vi "Measure Current.vi"(8 "error in":errorcluster, 11 "4124 in":refnum<class "4124.lvclass">) -> (0 "error out":errorcluster, 2 "Current":dbl, 3 "4124 out":refnum<class "4124.lvclass">)   [LabVIEW 2018, in "4124.lvlib" / "4124.lvclass"]
uses:
  4124.lvclass
  <instrlib>/NI RMX-412x Power Supplies/NI RMX-412x Power Supplies.lvlib
  builds/Power_Supply.lvlibp/Power Supply.lvclass
  C:/Users/Ron.Dexter.LUMINARTECH/Desktop/builds/Power_Supply.lvlibp/Power Supply.lvclass
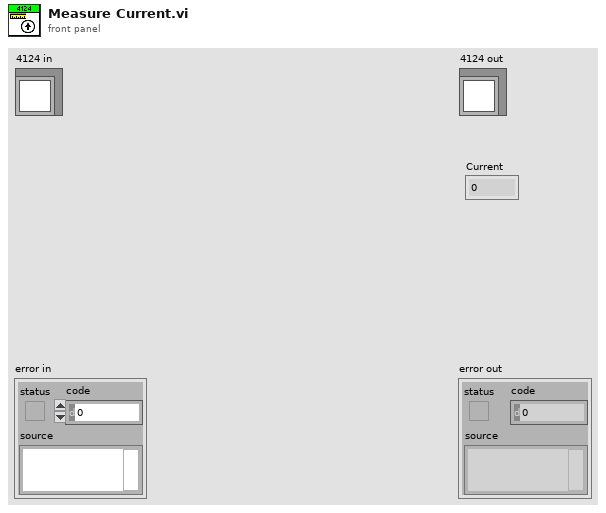
[diagram p1: front panel]
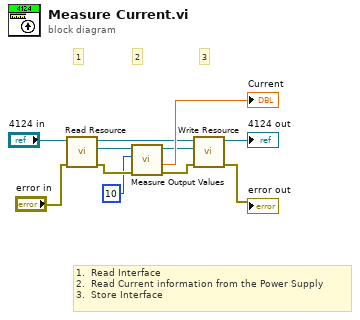
[diagram p0: block diagram]
diagram:
  # "1.  Read Interface\n2.  Read Current information from the Power Supply\n3.  Store Interface"
  # "3"
  # "2"
  # "1"
  n1 = call "Read Resource.vi"("error in"="error in", "Power Supply in"="4124 in") -> ("error out"=w7:errorcluster, "Resource"=w8:refnum<visa-resource-name>, "Power Supply out"=w6:refnum<class "4124.lvclass">)  [unwired: 7 in]
  n2 = call <instrlib>:"Measure Output Values.vi"("error in (no error)"=w7, "Wait Before Query (1550 ms)"=u32 10, "VISA resource name"=w8) -> ("error out"=w3:errorcluster, "Current Output"=→"Current":dbl, "VISA resource name out"=w4:refnum<visa-resource-name>)  [unwired: 5 in, 1 out]
  n3 = call "Write Resource.vi"("error in"=w3, "Resource"=w4, "Power Supply in"=w6) -> ("error out"=→"error out":errorcluster, "Power Supply out"=→"4124 out":refnum<class "4124.lvclass">)  [unwired: 7 in]
